vi "Switch-Selected Autonomous Example.vi"() -> ()   [LabVIEW 2016]
panel:
  out "DIP Switches":bool[](array[boolean])
  in  "stop":bool
  # "This example reads the state of the four DIP Switches on the Huskie Board  (D1, D2, D3, D4) and reflects their state in these boolean indicators. The indicators are updated while the VI runs so changes to the DIP switches are reflected as they are made.\n\nThese DIP switches are a reliable way to set the autonomous mode on the field. This example can be used to reflect the field-selected autonomous mode on the Driver Station.\n\nThe state of the DIP switches is also reflected in the corresponding LEDs on the Huskie Board for visual feedback."
  # "1"
  # "2"
  # "3"
  # "4"
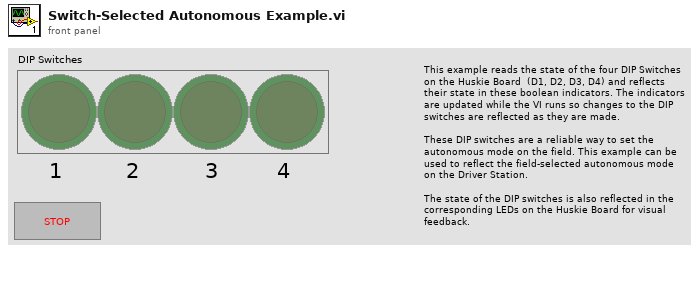
[diagram p1: front panel]
types:
  T1 = typedef "WPI_SerialPortRef.ctl" = cluster{"DevStatus":errorcluster, "Serial Port Name":refnum<visa-resource-name>}
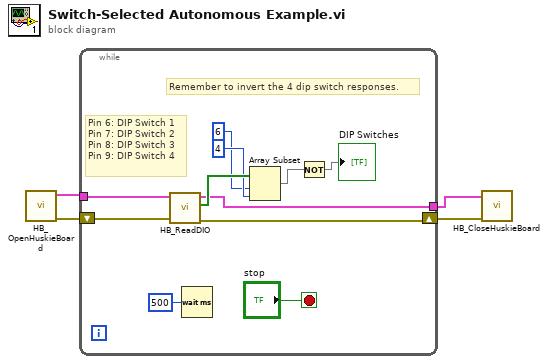
[diagram p0: block diagram]
diagram:
  n1 = call <vilib>:"HB_OpenHuskieBoard.vi"() -> ("error out"=w4:errorcluster, "HBDeviceRef"=w3:T1)  [unwired: 10 in]
  n2 = while {
    shift-right: [w11] -> w2
    shift-left: w4 -> [w12]
    tunnel: w3 -> [w13]
    tunnel: [w7] -> w1
    stop <- "stop" stop-if-true
    # "Remember to invert the 4 dip switch responses."
    # "Pin 6: DIP Switch 1\nPin 7: DIP Switch 2\nPin 8: DIP Switch 3\nPin 9: DIP Switch 4"
    n3 = call <vilib>:"HB_ReadDIO.vi"("error in (no error)"=w12, "HBDeviceRef"=w13) -> ("error out"=w11:errorcluster, "All Digital Input Vals"=w10:bool[], "HBDeviceRef"=w7:T1)  [unwired: 7 in]
    n4 = Wait (ms)(milliseconds to wait=u32 500) -> ()  [unwired: 1 out]
    n5 = Array Subset(array=w10, index=6, length=4) -> (w6:bool[])
    n6 = Not(x=w6) -> (.not. x?=→"DIP Switches":bool[])
  }
  n7 = call <vilib>:"HB_CloseHuskieBoard.vi"("error in (no error)"=w2, "HBDeviceRef"=w1) -> ()  [unwired: 9 in, 1 out]
